vi "CompressImagesToAvi.vi"() -> ()   [LabVIEW 2013]
panel:
  out "stop timer":bool
  out "seconds":dbl
  out "Numeric":i32
  in  "Frames Per Second":u32=30
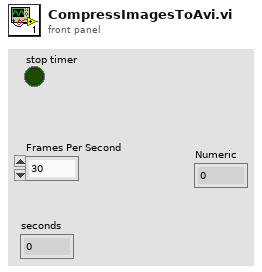
[diagram p1: front panel]
types:
  T1 = typedef "Image Type" = u32
  T2 = typedef "IMAQ AVI2 Refnum.ctl" = refnum<k20>
  T3 = typedef "IMAQ Image.ctl" = refnum<image>
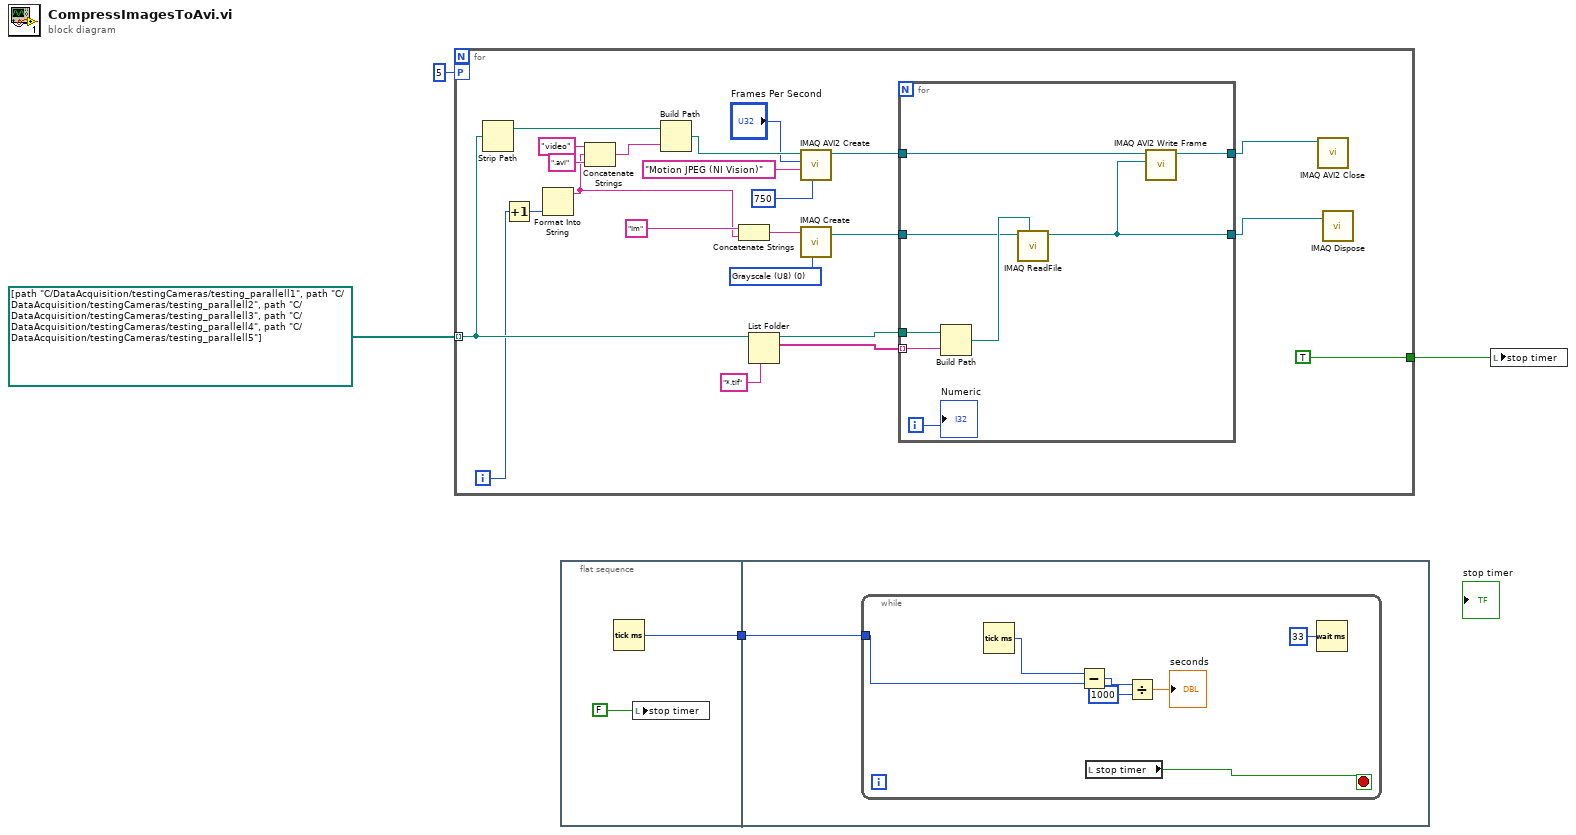
[diagram p0: block diagram]
diagram:
  n1 = for {
    tunnel: path[] [path "C:/DataAcquisition/testingCameras/testing_parallell1", path "C:/DataAcquisition/testingCameras/testing_parallell2", path "C:/DataAcquisition/testingCameras/testing_parallell3", path "C:/DataAcquisition/testingCameras/testing_parallell4", path "C:/DataAcquisition/testingCameras/testing_parallell5"] -> [w13] mode=indexing
    tunnel: [TRUE] -> w2
    workers-P: 5 -> [_]
    i -> [w8]
    w26 = T1 0 items=["Grayscale (U8)", "Grayscale (I16)", "Grayscale (SGL)", "Complex (CSG)", "RGB (U32)", "HSL (U32)", "RGB (U64)", "Grayscale (U16)"] ("Image Type")
    n2 = Strip Path(path=w13) -> (stripped path=w12:path)  [unwired: 1 out]
    n3 = Increment(x=w8) -> (x+1=w9:i32)
    n4 = Format Into String(w9) -> (resulting string=w6:string)  [unwired: 3 in, 1 out]
    n5 = Concatenate Strings("video" ("string"), w6, ".avi" ("string")) -> (w19:string)
    n6 = Build Path(base path=w12, name or relative path=w19) -> (appended path=w24:path)
    n7 = Concatenate Strings("Im" ("Image Name"), w6) -> (w5:string)
    n8 = List Folder(path=w13, pattern="*.tif") -> (path out=w17:path, filenames=w16:string[])  [unwired: 2 in, 2 out]
    n9 = call "IMAQ AVI2 Create"("Quality"=750, "Codec"="Motion JPEG (NI Vision)", "Frames Per Second"="Frames Per Second", "AVI Path"=w24) -> ("AVI Refnum"=w18:T2)  [unwired: 6 in, 1 out]
    n10 = call "IMAQ Create"("Image Name"=w5, "Image Type"=w26) -> ("New Image"=w15:T3)  [unwired: 3 in, 1 out]
    n11 = for {
      tunnel: w18 -> [w35]
      tunnel: [w32] -> w11
      tunnel: [w31] -> w10
      tunnel: w17 -> [w30]
      tunnel: w16 -> [w29] mode=indexing
      tunnel: w15 -> [w28]
      i -> [w33]
      n12 = Build Path(base path=w30, name or relative path=w29) -> (appended path=w34:path)
      n13 = call "IMAQ ReadFile"("File Path"=w34, "Image"=w28) -> ("Image Out"=w31:T3)  [unwired: 5 in, 4 out]
      n14 = call "IMAQ AVI2 Write Frame"("Image"=w31, "AVI Refnum"=w35) -> ("AVI Refnum (duplicate)"=w32:T2)  [unwired: 7 in, 2 out]
      "Numeric" <- w33
    }
    n15 = call "IMAQ AVI2 Close"("AVI Refnum"=w11) -> ()  [unwired: 10 in, 1 out]
    n16 = call "IMAQ Dispose"("Image"=w10) -> ()  [unwired: 5 in, 1 out]
  }
  n17 = flat-sequence {
    tunnel: [w37] -> w4
    tunnel: w4 -> [w38]
    frame #0 {
      n18 = Tick Count (ms)() -> (millisecond timer value=w37:u32)
      n19 = local write "stop timer"(FALSE) -> ()
    }
    frame #1 {
      n20 = while {
        tunnel: w38 -> [w39]
        stop <- w40 stop-if-true
        n21 = Tick Count (ms)() -> (millisecond timer value=w44:u32)
        n22 = Subtract(x=w44, y=w39) -> (x-y=w43:u32)
        n23 = local read "stop timer"() -> (w40:bool)
        n24 = Divide(x=w43, y=u32 1000) -> (x/y=→"seconds":dbl)
        n25 = Wait (ms)(milliseconds to wait=u32 33) -> ()  [unwired: 1 out]
      }
    }
  }
  n26 = local write "stop timer"(w2) -> ()
